vi "Write Error Log Entry.vi"(7 "Classification":T1, 8 "error in (no error)":errorcluster, 9 "base path":path, 10 "current time":timestamp, 11 "Section of System":string caption="Account #") -> (0 "error out":errorcluster)   [LabVIEW 2024]
uses:
  Controls/Error Classification.ctl
  <vilib>/Utility/error.llb/DialogType.ctl
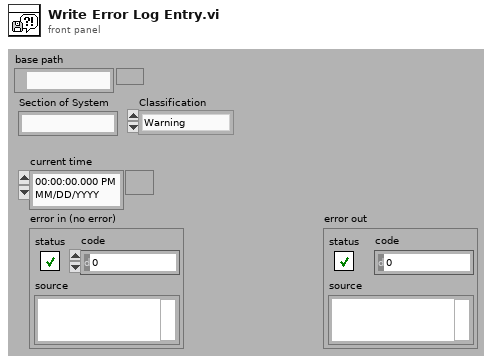
[diagram p1: front panel]
types:
  T1 = typedef "Error Classification.ctl" = enum16{"Warning", "Non-Critical", "Critical"}
  T2 = enum16{"open", "replace", "create", "open or create", "replace or create", "replace or create with confirmation"}
  T3 = typedef "DialogType.ctl" = u16
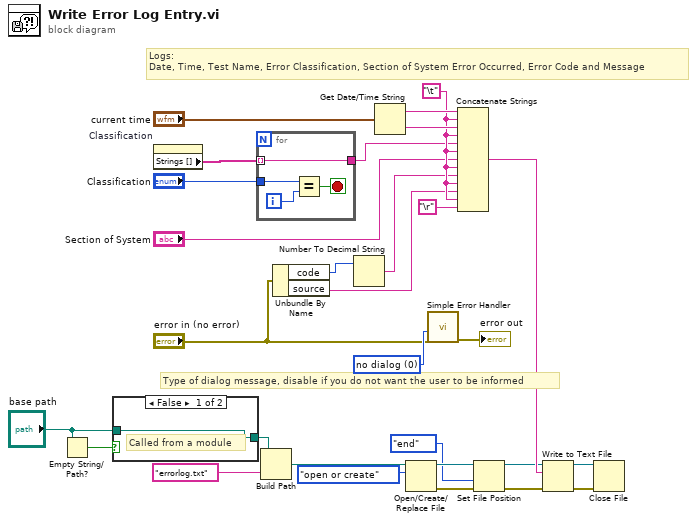
[diagram p0: block diagram]
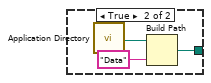
[diagram p2: hidden frame]
diagram:
  w15 = "\t"
  w28 = T3 0 items=["no dialog", "OK message", "continue or stop message", "OK message + warnings", "continue/stop + warnings"] ("type of dialog (OK msg:1)")
  # "Logs:\nDate, Time, Test Name, Error Classification, Section of System Error Occurred, Error Code and Message"
  # "Type of dialog message, disable if you do not want the user to be informed"
  n1 = Empty String/Path?(string/path="base path") -> (empty?=w2:bool)
  n2 = case shown="False" w2 {
    tunnel: [w30 w33] -> w18
    tunnel: "base path" -> [w30 _]
    frame False {
      # "Called from a module"
    }
    frame True {
      n3 = call <vilib>:"Application Directory.vi"() -> ("Application Directory"=w31:path)
      n4 = Build Path(base path=w31, name or relative path="Data") -> (appended path=w33:path)
    }
  }
  n5 = property on="Classification" class="Enum (strict)"() -> ("Strings []"=w22:string[])  [unwired: 2 in, 2 out]
  n6 = for {
    tunnel: "Classification" -> [w36]
    tunnel: [w35] -> w12
    tunnel: w22 -> [w35] mode=indexing
    i -> [w37]
    stop <- w34 stop-if-true
    n7 = Equal?(x=w36, y=w37) -> (x = y?=w34:bool)
  }
  n8 = Build Path(base path=w18, name or relative path="errorlog.txt") -> (appended path=w21:path)
  n9 = Unbundle By Name("error in (no error)") -> ("code"=w25:i32, "source"=w9:string)
  n10 = Number To Decimal String(number=w25) -> (decimal integer string=w10:string)  [unwired: 1 in]
  n11 = Get Date/Time String(seconds (now)="current time") -> (date string=w27:string, time string=w26:string)  [unwired: 2 in]
  n12 = Open/Create/Replace File(file path (use dialog)=w21, operation (0:open)=T2."open or create") -> (refnum out=w5:refnum<file>, error out=w7:errorcluster)  [unwired: 4 in, 1 out]
  n13 = call <vilib>:"Simple Error Handler.vi"("type of dialog (OK msg:1)"=w28, "error in (no error)"="error in (no error)") -> ("error out"=→"error out":errorcluster)  [unwired: 3 in, 4 out]
  n14 = Concatenate Strings(w27, w15, w26, w15, w12, w15, "Section of System", w15, w10, w15, w9, w15, "\r") -> (w14:string)
  n15 = Set File Position(refnum=w5, from (0:start)=enum16{"start", "end", "current"}."end", error in=w7) -> (refnum out=w4:refnum<file>, error out=w6:errorcluster)  [unwired: 1 in]
  n16 = Write to Text File(file (use dialog)=w4, text=w14, error in=w6) -> (refnum out=w16:refnum<file>, error out=w17:errorcluster)  [unwired: 1 in, 1 out]
  n17 = Close File(refnum=w16, error in=w17) -> ()  [unwired: 2 out]
